vi "FPGA_digitizer_range_test.vi"() -> ()   [LabVIEW 2012]
uses:
  <vilib>/Platform/TimedLoop/XDataNode/XDataNode.xnode
  <vilib>/Platform/TimedLoop/XDataNode/nitl_modes.ctl
  <vilib>/Platform/TimedLoop/XDataNode/XDNodeRunTimeDep.lvlib
  <vilib>/Platform/TimedLoop/XDataNode/wakeup.ctl
  <vilib>/Platform/TimedLoop/XDataNode/timing_clust.ctl
  <vilib>/rvi/DataTransferAndStorage/Container/XNode/niFpgaContainer.xnode
  <vilib>/eio/EIONode/EIONode.xnode
  <vilib>/rvi/eio/common/nirviEmuTemplateMethod_errors.vi
  <vilib>/rvi/FIFO/Fifo_Resource/nirvififoEmulationWrite.vi
panel:
  out "IO Module\\Pll Unlocked":bool
  out "IO Module\\ADC Error B":bool
  out "IO Module\\ADC Error A":bool
  out "Init Done":bool
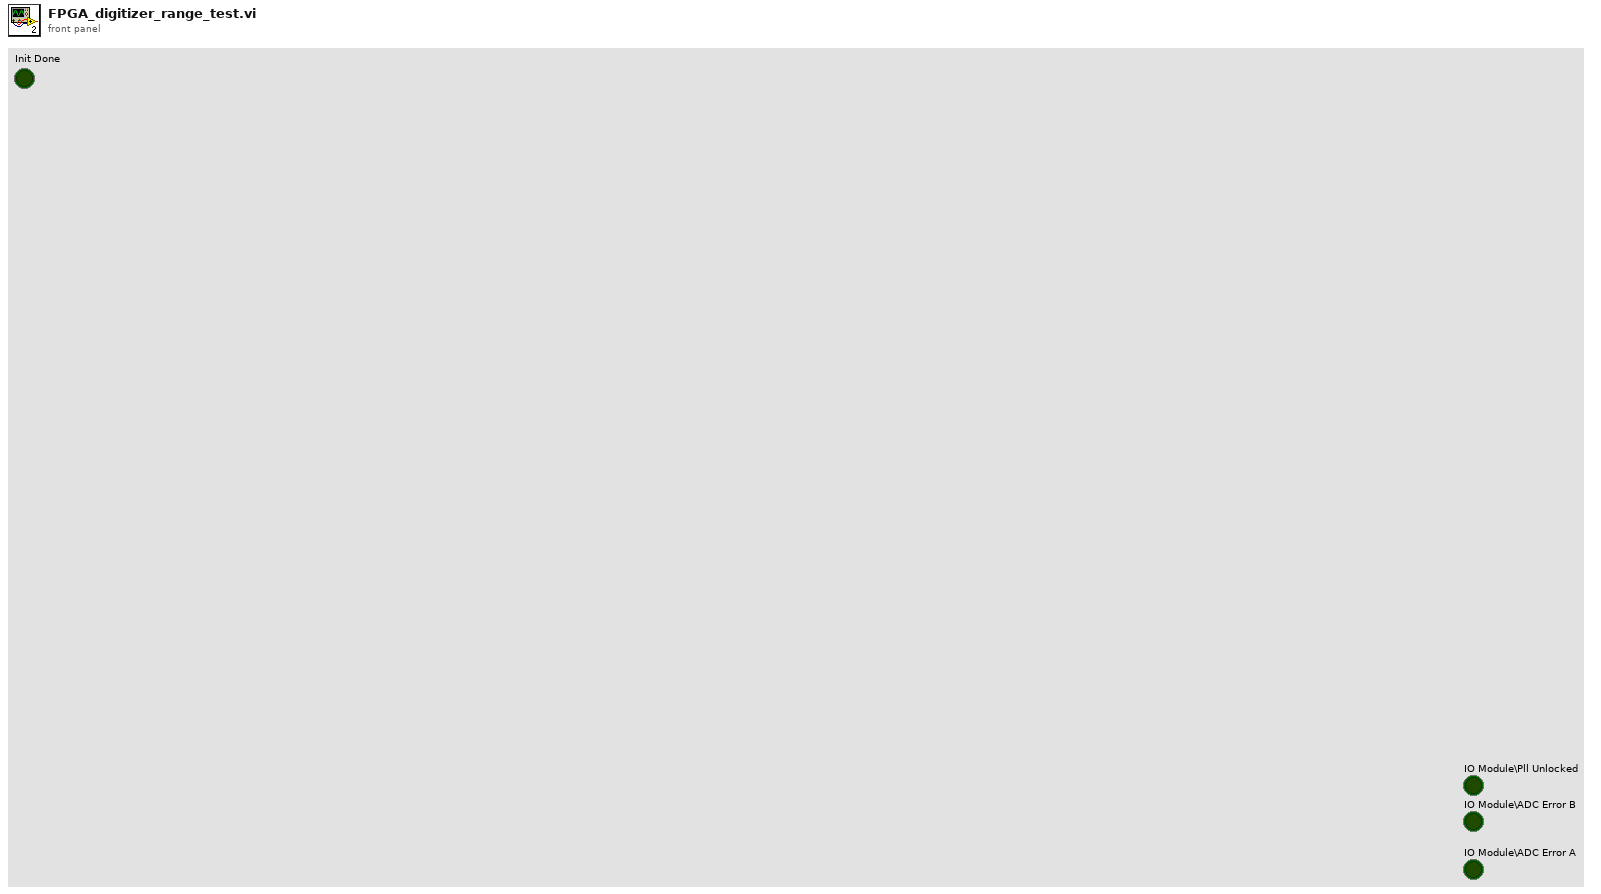
[diagram p1: front panel]
types:
  T1 = typedef "XDNodeRunTimeDep.lvlib/timing_clust.ctl" = cluster{"Expected End [f-1]":u64, "Actual End [f-1]":u64, "Finished Late? [f-1]":bool, "Expected End [i-1]":u64, "Actual End [i-1]":u64, "Finished Late? [i-1]":bool, "Expected Start [i]":u64, "Actual Start [i]":u64, "Expected Start [f]":u64, "Actual Start [f]":u64, "Source Name":string, "Structure Name":string, "Period":i64, "Deadline":i64, "Offset":i64, "Start":i64, "Priority":i32, "Timeout":i32, "Mode":T2, "Wakeup Reason":T3, "Error":errorcluster, "Source Type":string, "Secondary Source Type":string, "Global End Time":u64, "Global Start Time":u64, "Frame Duration":u64, "Iteration Duration":u64, "Assigned CPU":i32, "I/O Scan Engine Mode":u32}
  T2 = typedef "XDNodeRunTimeDep.lvlib/nitl_modes.ctl" = enum32{"No Change", "Process missed periods, maintain original phase", "Discard missed periods, maintain original phase", "Process missed periods, ignore original phase", "Discard missed periods, ignore original phase"}
  T3 = typedef "XDNodeRunTimeDep.lvlib/wakeup.ctl" = enum32{"Normal", "Aborted", "Asynchronous wakeup", "Timing source error", "Timed loop error", "Timeout"}
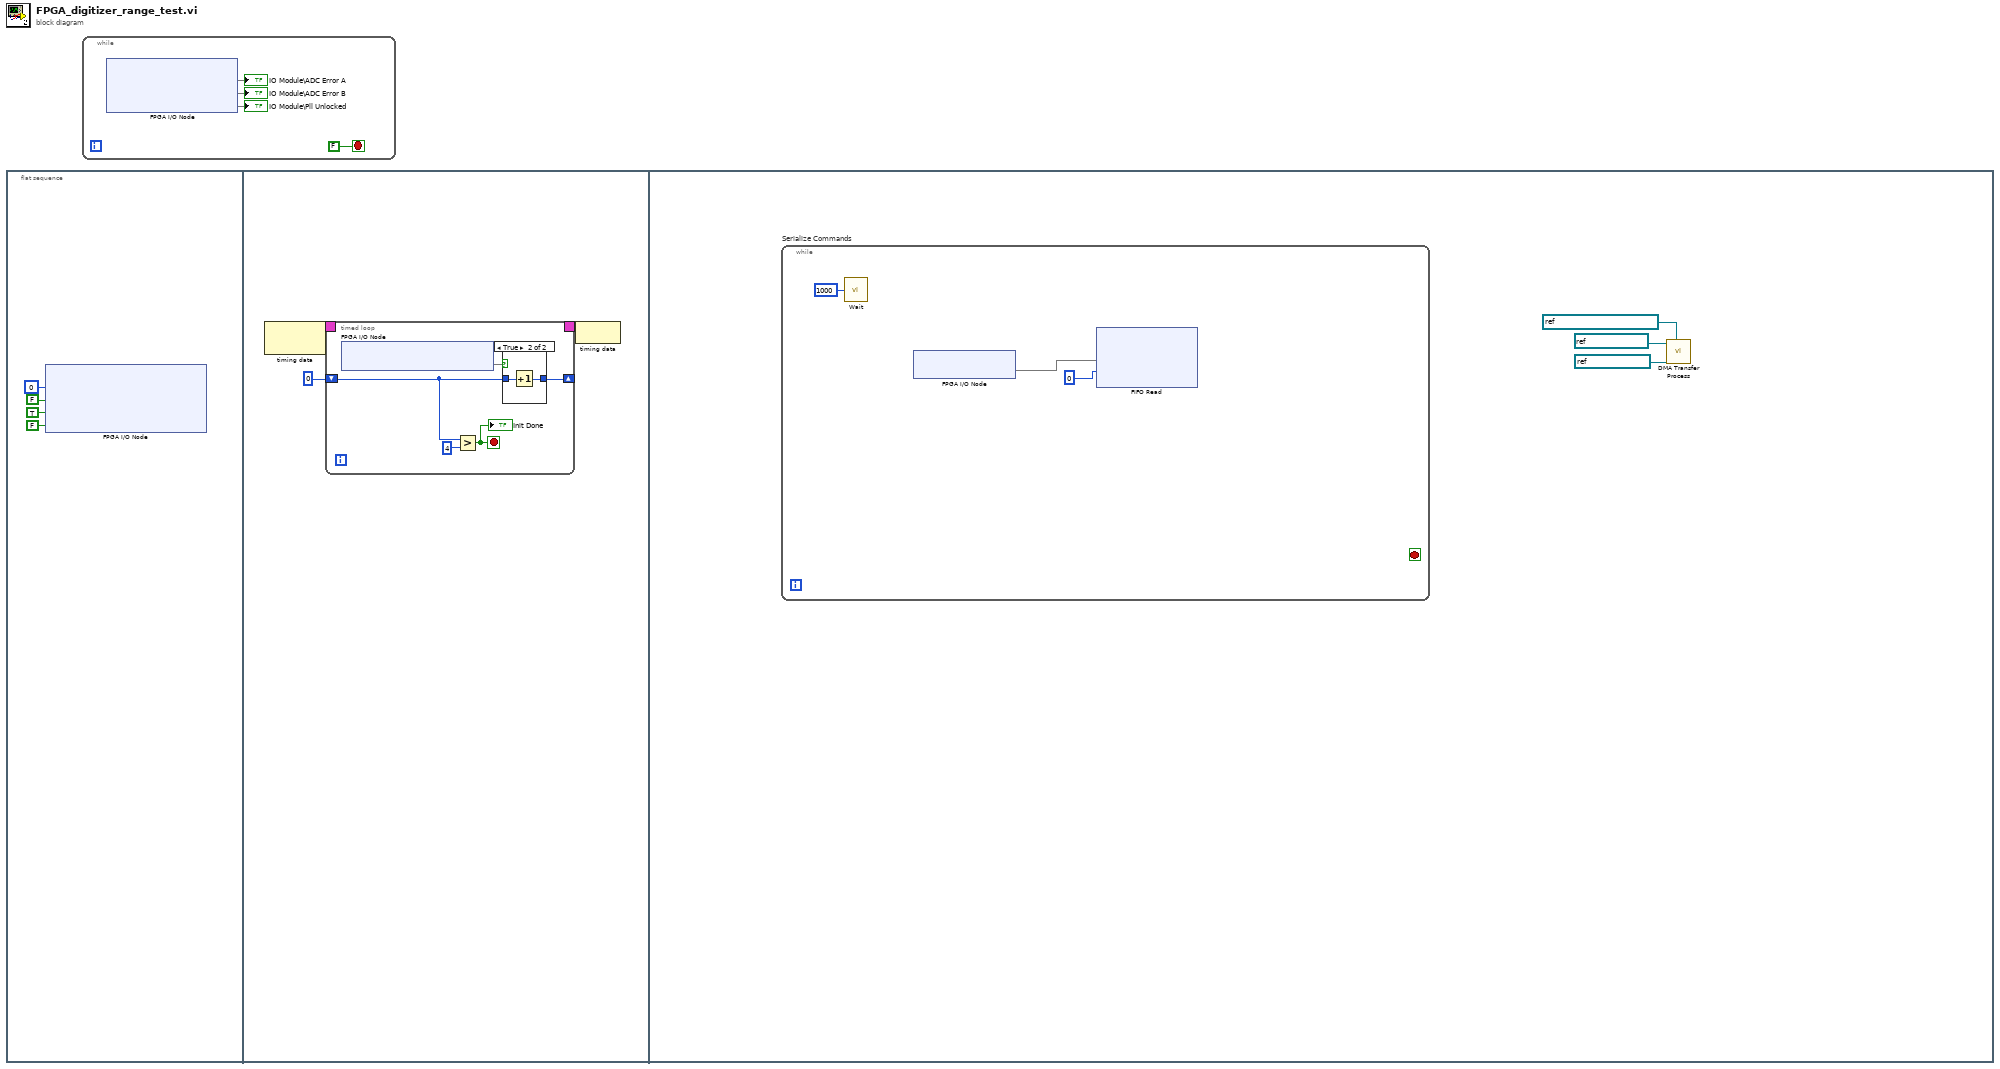
[diagram p0: block diagram]
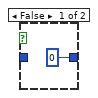
[diagram p2: hidden frame]
diagram:
  n1 = flat-sequence {
    frame #0 {
      n2 = xnode "FPGA I/O Node"("IO Module\\Sample Clock Select"=u8 0 ("IO Module\\Sample Clock Select"), "IO Module\\Force Initialization"=FALSE ("IO Module\\Force Initialization"), "IO Module\\Force Initialization"=TRUE ("IO Module\\Force Initialization"), "IO Module\\Force Initialization"=FALSE ("IO Module\\Force Initialization")) -> ()  [unwired: 4 in, 4 out]
    }
    frame #1 {
      n3 = node-c288() -> (w7:T1)  [unwired: 1 in]
      n4 = timed-loop {
        shift-right: [w11] -> _
        shift-left: u16 0 -> [w10]
        timing: w7 -> [_]
        timing-out: [_] -> w6
        stop <- w8 stop-if-true
        n5 = xnode "FPGA I/O Node"() -> ("IO Module\\Initialization Done"=w12)  [unwired: 1 in, 1 out]
        n6 = Greater?(x=w10, y=u16 4) -> (0:w8:bool)
        "Init Done" <- w8
        n7 = case shown="True" w12 {
          tunnel: [u16 0 w15] -> w11
          tunnel: w10 -> [_ w14]
          frame False {
          }
          frame True {
            n8 = Increment(x=w14) -> (x+1=w15:u16)
          }
        }
      }
      n9 = node-c288(w6) -> ()
    }
    frame #2 {
      n10 = while "Serialize Commands" {
        stop <- _ stop-if-true
        n11 = call "Wait"("Count(uSec)"=u32 1000) -> ()  [unwired: 1 out]
        n12 = xnode "FPGA I/O Node"() -> ("IO Module\\AI A0"=w24)  [unwired: 1 in, 1 out]
        n13 = xnode ("FIFO Read")("Element"=w24, "Timeout"=0) -> ()  [unwired: 1 in, 2 out]
      }
      n14 = call "DMA Transfer Process.vi"("Clock Domain"=refnum<k21> "40 MHz Onboard Clock", "Local"=refnum<k21> "To DMA FIFO", "DMA"=refnum<k21> "To Host FIFO") -> ()  [unwired: 9 in]
    }
  }
  n15 = while {
    stop <- FALSE stop-if-true
    n16 = xnode "FPGA I/O Node"() -> ("IO Module\\ADC Error A"=→"IO Module\\ADC Error A", "IO Module\\ADC Error B"=→"IO Module\\ADC Error B", "IO Module\\Pll Unlocked"=→"IO Module\\Pll Unlocked")  [unwired: 3 in, 3 out]
  }
